vi "EXPORT DATA.vi"() -> ()   [LabVIEW 2015]
uses:
  <vilib>/addons/database/Connection.llb/DB Tools Open Connec (Path).vi
  <vilib>/addons/database/Connection.llb/Conn Execute.vi
  <vilib>/addons/database/Recordset.llb/Rec Fetch Recordset Data (R).vi
  <vilib>/addons/database/Recordset.llb/Rec Destroy - Connection.vi
  <vilib>/addons/database/NI_Database_API.lvlib
panel:
  out "error out":errorcluster
  out "resulting string":string
  out "Array":string[][](array[string])
  in  "date string":string
  in  "invoid":string
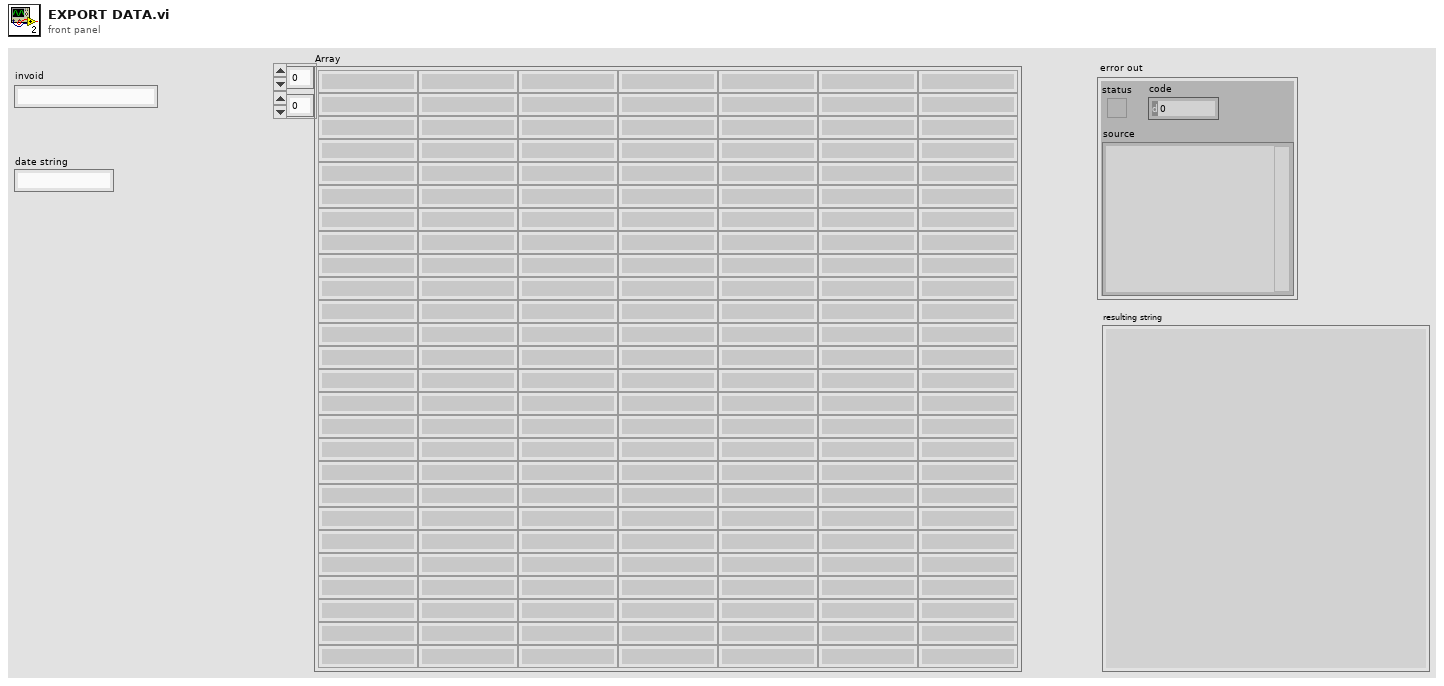
[diagram p1: front panel]
types:
  T1 = typedef "NI_Database_API.lvlib/Conn ObjectReference.ctl" = refnum<k1>
  T2 = typedef "NI_Database_API.lvlib/Rec ObjectReference.ctl" = refnum<k1>
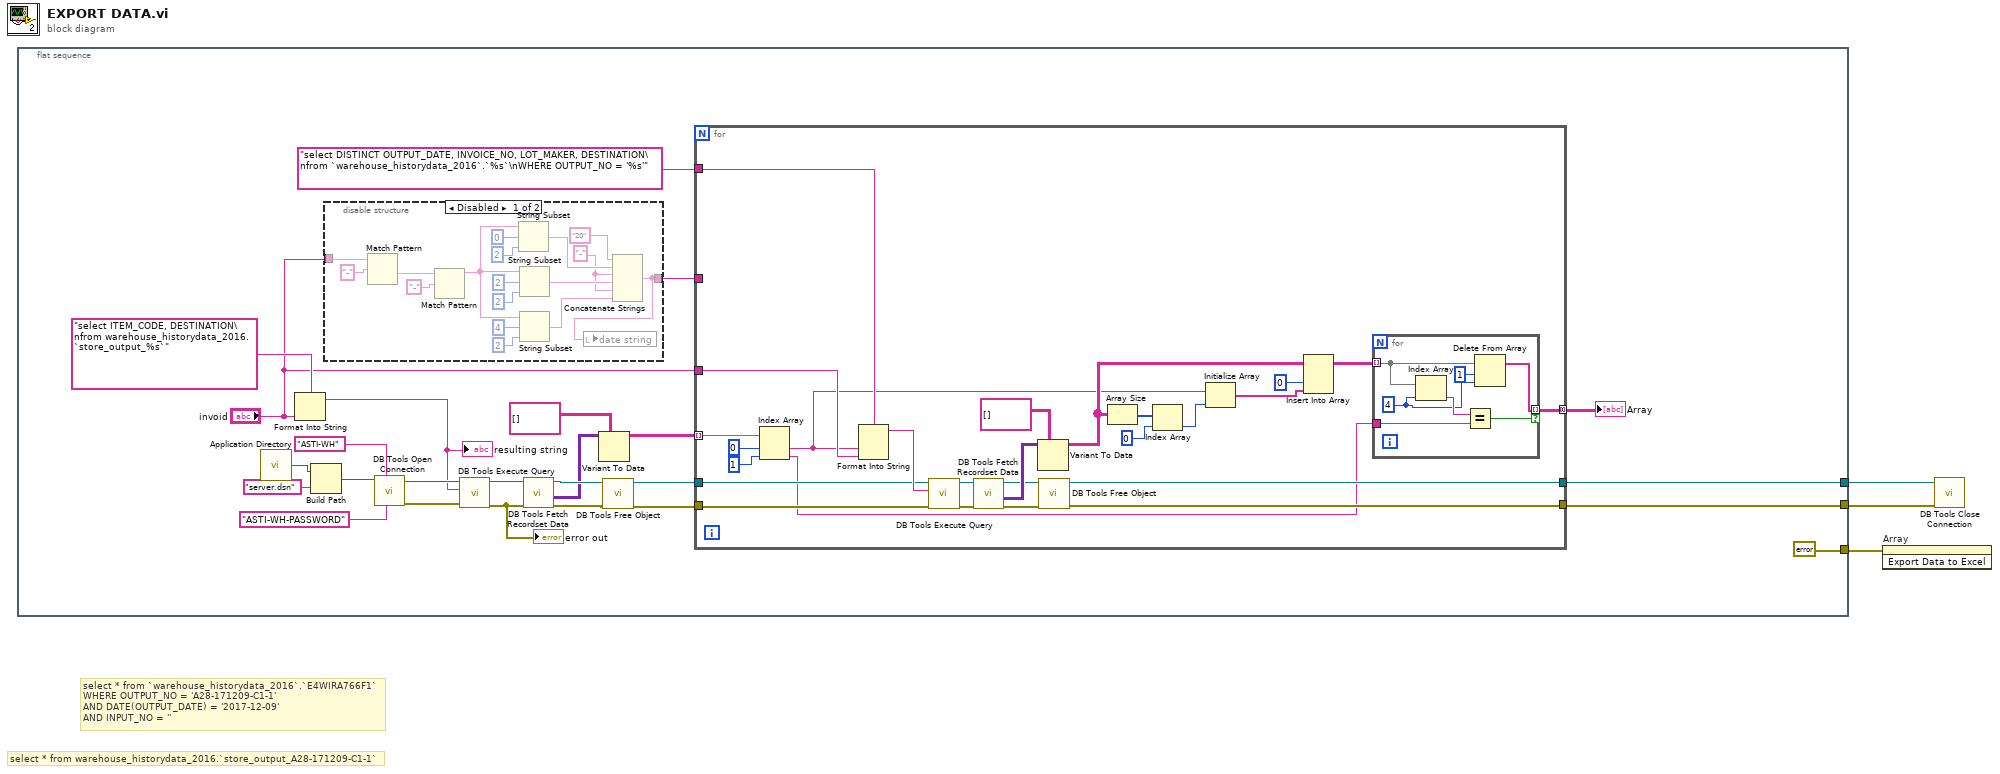
[diagram p0: block diagram]
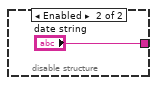
[diagram p2: hidden frame]
diagram:
  # "select * from warehouse_historydata_2016.`store_output_A28-171209-C1-1`"
  # "select * from `warehouse_historydata_2016`.`E4WIRA766F1`\nWHERE OUTPUT_NO = 'A28-171209-C1-1'\nAND DATE(OUTPUT_DATE) = '2017-12-09'\nAND INPUT_NO = ''"
  n1 = flat-sequence {
    tunnel: [errorcluster {"status"=FALSE, "code"=0, "source"=""} ("error constant")] -> w3
    tunnel: [w5] -> w2
    tunnel: [w4] -> w1
    frame #0 {
      n2 = call <vilib>:"Application Directory.vi"() -> ("Application Directory"=w26:path)
      n3 = Format Into String(format string="select ITEM_CODE, DESTINATION\nfrom warehouse_historydata_2016.`store_output_%s`", "invoid") -> (resulting string=w20:string)  [unwired: 2 in, 1 out]
      "resulting string" <- w20
      n4 = Build Path(base path=w26, name or relative path="server.dsn") -> (appended path=w24:path)
      n5 = disable-structure shown="Disabled" {
        disable-tunnel: "invoid" -> [w45 _]
        disable-tunnel: [w29 "date string"] -> w10
        frame Disabled {
          w31 = "-" ("string")
          n6 = Match Pattern(string=w45, regular expression="-" ("search string")) -> (after substring=w42:string)  [unwired: 1 in, 3 out]
          n7 = Match Pattern(string=w42, regular expression="-" ("search string")) -> (before substring=w35:string)  [unwired: 1 in, 3 out]
          n8 = String Subset(string=w35, offset (0)=0, length (rest)=2 ("length (rest)")) -> (substring=w33:string)
          n9 = String Subset(string=w35, offset (0)=2, length (rest)=2 ("length (rest)")) -> (substring=w32:string)
          n10 = String Subset(string=w35, offset (0)=4, length (rest)=2 ("length (rest)")) -> (substring=w30:string)
          n11 = Concatenate Strings("20", w33, w31, w32, w31, w30) -> (w29:string)
          n12 = local write "date string"(w29) -> ()
        }
        frame Enabled {
        }
      }
      n13 = call-poly <vilib>:"DB Tools Open Connection.vi"("password"="ASTI-WH-PASSWORD", "userID"="ASTI-WH", "connection information"=w24) -> ("error out"=w22:errorcluster, "connection reference"=w23:T1)  [unwired: 5 in]
      n14 = call-poly <vilib>:"DB Tools Execute Query.vi"("error in (no error)"=w22, "SQL query"=w20, "connection reference"=w23) -> ("error out"=w18:errorcluster, "recordset reference"=w19:T2)  [unwired: 5 in]
      "error out" <- w18
      n15 = call-poly <vilib>:"DB Tools Fetch Recordset Data.vi"("error in (no error)"=w18, "recordset reference"=w19) -> ("error out"=w16:errorcluster, "recordset data"=w15:variant[][], "recordset reference out"=w17:T2)  [unwired: 3 in]
      n16 = Variant To Data(type=string[][] [], Variant=w15) -> (data=w13:string[][])  [unwired: 1 in, 1 out]
      n17 = call-poly <vilib>:"DB Tools Free Object.vi"("error in (no error)"=w16, "recordset reference"=w17) -> ("error out"=w8:errorcluster, "connection reference"=w9:T1)  [unwired: 8 in]
      n18 = for {
        tunnel: w13 -> [w57] mode=indexing
        tunnel: "select DISTINCT OUTPUT_DATE, INVOICE_NO, LOT_MAKER, DESTINATION\nfrom `warehouse_historydata_2016`.`%s`\nWHERE OUTPUT_NO = '%s'" -> [w66]
        tunnel: "invoid" -> [w65]
        tunnel: w10 -> [_]
        tunnel: w9 -> [w63]
        tunnel: w8 -> [w62]
        tunnel: [w47] -> w7 mode=concatenating
        tunnel: [w61] -> w5
        tunnel: [w60] -> w4
        n19 = Index Array(array=w57, index #1=0 ("disabled index (col)"), index #2=1 ("disabled index (col)")) -> (element #1=w52:string, element #2=w49:string)
        n20 = Format Into String(format string=w66, w52, w65) -> (resulting string=w64:string)  [unwired: 2 in, 1 out]
        n21 = call-poly <vilib>:"DB Tools Execute Query.vi"("error in (no error)"=w62, "SQL query"=w64, "connection reference"=w63) -> ("error out"=w68:errorcluster, "recordset reference"=w67:T2)  [unwired: 5 in]
        n22 = call-poly <vilib>:"DB Tools Fetch Recordset Data.vi"("error in (no error)"=w68, "recordset reference"=w67) -> ("error out"=w70:errorcluster, "recordset data"=w71:variant[][], "recordset reference out"=w69:T2)  [unwired: 3 in]
        n23 = Variant To Data(type=string[][] [], Variant=w71) -> (data=w53:string[][])  [unwired: 1 in, 1 out]
        n24 = call-poly <vilib>:"DB Tools Free Object.vi"("error in (no error)"=w70, "recordset reference"=w69) -> ("error out"=w60:errorcluster, "connection reference"=w61:T1)  [unwired: 8 in]
        n25 = Array Size(array=w53) -> (size(s)=w59:i32[])
        n26 = Index Array(array=w59, index=0) -> (element=w56:i32)
        n27 = Initialize Array(w52, w56) -> (w54:string[])
        n28 = Insert Into Array(array=w53, index (col)=0 ("disabled index (col)"), new element=w54) -> (w48:string[][])  [unwired: 1 in]
        n29 = for {
          tunnel: w49 -> [w79]
          tunnel: [w75] -> w47 mode=indexing if=w78
          tunnel: w48 -> [w76] mode=indexing
          w74 = 4 ("index (col)")
          n30 = Index Array(array=w76, index=w74) -> (element=w77:string)
          n31 = Equal?(x=w77, y=w79) -> (x = y?=w78:bool)
          n32 = Delete From Array(array=w76, length=1, index=w74) -> (array with subset deleted=w75:string[])  [unwired: 1 out]
        }
      }
      "Array" <- w7
    }
  }
  n33 = invoke on="Array" class="Arr (strict)" method="Export Data to Excel"(error in=w3) -> ()  [unwired: 2 in, 3 out]
  n34 = call <vilib>:"DB Tools Close Connection.vi"("error in (no error)"=w1, "connection reference"=w2) -> ()  [unwired: 5 in, 1 out]
